vi "Wave Mask.vi"(8 "error in (no error)":errorcluster, 10 "signal type":T1(ring), 11 "Queue in":refnum<queue>) -> (0 "error out":errorcluster, 1 "error out 3":errorcluster, 2 "error out 2":errorcluster, 3 "test passed?":bool, 5 "output values":waveform(dbl)[](array[waveform]))   [LabVIEW 2016]
uses:
  <vilib>/measure/mamon.llb/Create Continuous Mask.vi
  <vilib>/measure/mamon.llb/Limit Testing Time.vi
  <vilib>/measure/matone.llb/Extract Single Tone Information 1 Chan.vi
  <vilib>/measure/NI_MAPro.lvlib
  <vilib>/measure/NI_MABase.lvlib
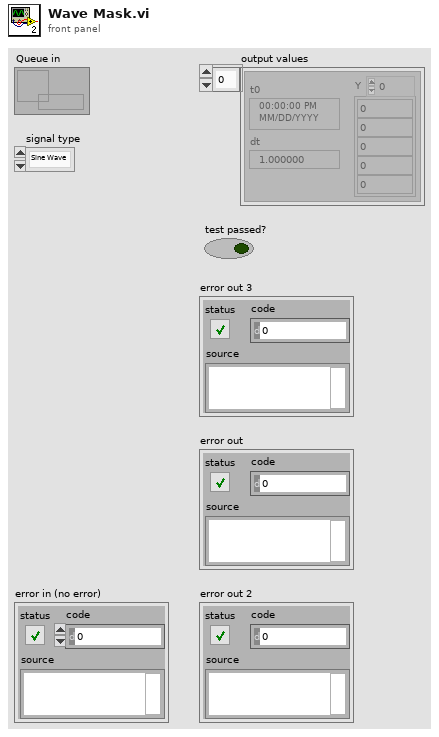
[diagram p1: front panel]
types:
  T1 = enum16{"Sine Wave", "Triangle Wave", "Square Wave", "Sawtooth Wave"}
  T2 = cluster{"pass region":i32, "include UL":bool, "include LL":bool}
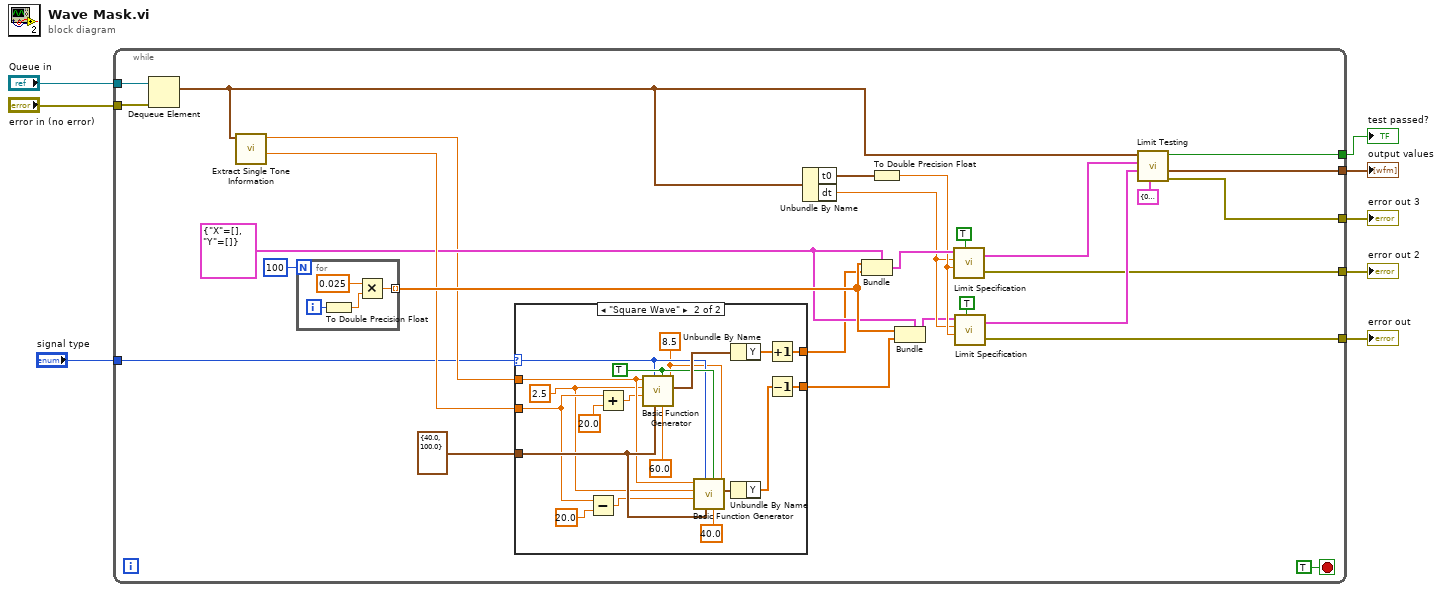
[diagram p0: block diagram]
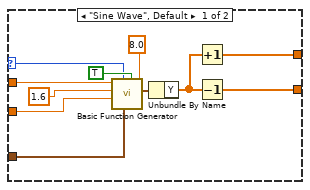
[diagram p2: hidden frame]
diagram:
  n1 = while {
    tunnel: "Queue in" -> [w36]
    tunnel: "error in (no error)" -> [w35]
    tunnel: "signal type" -> [w15]
    tunnel: [w14] -> w4
    tunnel: [w13] -> w5
    tunnel: [w12] -> w6
    tunnel: [w11] -> w7
    tunnel: [w10] -> w8
    stop <- TRUE stop-if-true
    w20 = cluster{"X":dbl[], "Y":dbl[]} {"X"=[], "Y"=[]} ("Specification Cluster")
    n2 = Dequeue Element(queue=w36, error in (no error)=w35) -> (element=w21:waveform(dbl))  [unwired: 1 in, 3 out]
    n3 = call-poly <vilib>:"Extract Single Tone Information.vi"("time signal in"=w21) -> ("detected phase (deg)"=w29:dbl, "detected frequency"=w19:dbl)  [unwired: 5 in, 4 out]
    n4 = for {
      N: 100 -> [_]
      tunnel: [w70] -> w31 mode=indexing
      i -> [w68]
      n5 = To Double Precision Float(number=w68) -> (double precision float=w67:dbl)
      n6 = Multiply(x=0.025 ("y"), y=w67) -> (x*y=w70:dbl)
    }
    n7 = case shown="\"Square Wave\"" w15 {
      selector: w15 -> [w42 w59]
      tunnel: cluster{"Fs":dbl, "#s":dbl} {"Fs"=40.0, "#s"=100.0} ("sampling info") -> [w47 w61]
      tunnel: w29 -> [w45 w50]
      tunnel: w19 -> [w43 w57]
      tunnel: [w40 w55] -> w17
      tunnel: [w38 w54] -> w16
      frame "Sine Wave", Default {
        n8 = call <vilib>:"Basic Function Generator.vi"("offset"=8.0, "reset signal"=TRUE, "sampling info"=w47, "signal type"=w42, "phase"=w45, "amplitude"=1.6, "frequency"=w43) -> ("signal out"=w41:waveform(dbl))  [unwired: 2 in, 2 out]
        n9 = Unbundle By Name(w41) -> ("Y"=w39:dbl[])
        n10 = Increment(x=w39) -> (x+1=w40:dbl[])
        n11 = Decrement(x=w39) -> (x-1=w38:dbl[])
      }
      frame "Square Wave" {
        w48 = 2.5 ("amplitude")
        w60 = TRUE ("reset signal")
        w58 = 8.5 ("offset")
        n12 = Subtract(x=w50, y=20.0) -> (x-y=w51:dbl)
        n13 = Add(x=w50, y=20.0) -> (x+y=w53:dbl)
        n14 = call <vilib>:"Basic Function Generator.vi"("offset"=w58, "square wave duty cycle (%)"=60.0 ("square wave duty cycle (%) up"), "reset signal"=w60, "sampling info"=w61, "signal type"=w59, "phase"=w53, "amplitude"=w48, "frequency"=w57) -> ("signal out"=w65:waveform(dbl))  [unwired: 1 in, 2 out]
        n15 = call <vilib>:"Basic Function Generator.vi"("offset"=w58, "square wave duty cycle (%)"=40.0 ("square wave duty cycle (%) down"), "reset signal"=w60, "sampling info"=w61, "signal type"=w59, "phase"=w51, "amplitude"=w48, "frequency"=w57) -> ("signal out"=w64:waveform(dbl))  [unwired: 1 in, 2 out]
        n16 = Unbundle By Name(w65) -> ("Y"=w63:dbl[])
        n17 = Unbundle By Name(w64) -> ("Y"=w62:dbl[])
        n18 = Increment(x=w63) -> (x+1=w55:dbl[])
        n19 = Decrement(x=w62) -> (x-1=w54:dbl[])
      }
    }
    n20 = Unbundle By Name(w21) -> ("t0"=w26:timestamp, "dt"=w24:dbl)
    n21 = Bundle(cluster=w20, "X"=w31, "Y"=w17) -> (w34:cluster{"X":dbl[], "Y":dbl[]})
    n22 = To Double Precision Float(number=w26) -> (double precision float=w25:dbl)
    n23 = Bundle(cluster=w20, "X"=w31, "Y"=w16) -> (w22:cluster{"X":dbl[], "Y":dbl[]})
    n24 = call-poly <vilib>:"Limit Specification.vi"("Specification Cluster"=w34, "dx"=w24, "x0"=w25, "Reset"=TRUE) -> ("Limit"=w28:cluster{"x0":dbl, "dx":dbl, "Y":dbl[]}, "error out"=w11:errorcluster)  [unwired: 1 in]
    n25 = call-poly <vilib>:"Limit Specification.vi"("Specification Cluster"=w22, "dx"=w24, "x0"=w25, "Reset"=TRUE) -> ("Limit"=w23:cluster{"x0":dbl, "dx":dbl, "Y":dbl[]}, "error out"=w10:errorcluster)  [unwired: 1 in]
    n26 = call-poly <vilib>:"Limit Testing.vi"("limit test config"=T2 {"pass region"=0, "include UL"=TRUE, "include LL"=TRUE}, "lower limit"=w23, "upper limit"=w28, "signal in"=w21) -> ("error out"=w12:errorcluster, "output values"=w14:waveform(dbl)[], "test passed?"=w13:bool)  [unwired: 2 in, 3 out]
  }
  "error out" <- w8
  "error out 2" <- w7
  "error out 3" <- w6
  "test passed?" <- w5
  "output values" <- w4
